vi "Send Get Notifiers.vi"(8 "error in (no error)":errorcluster, 10 "Reply Queue":refnum<queue>, 11 "Message Queue in":refnum<queue>) -> (0 "error out":errorcluster, 3 "Message Queue out":refnum<queue>)   [LabVIEW 2024, in "PID Loop.lvlib" / "Get Notifiers.lvclass"]
uses:
  Get Notifiers.lvclass
  Get Notifiers.lvclass/Get Notifiers.ctl
  C:/Users/uspoaotto/OneDrive - Oregon Tool/Desktop/working copies/helperLoop/src/OOQMH/Message/Message.lvclass
  C:/Users/uspoaotto/OneDrive - Oregon Tool/Desktop/working copies/helperLoop/src/PID Loop/Get Notifiers/Get Notifiers.lvclass
  OOQMH/Message/Message.lvclass
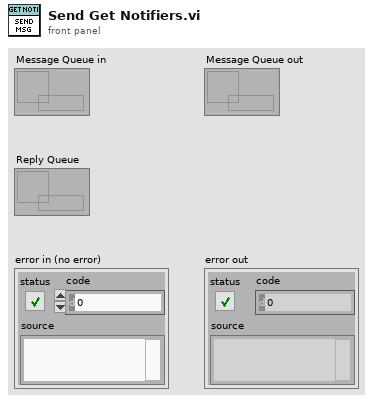
[diagram p1: front panel]
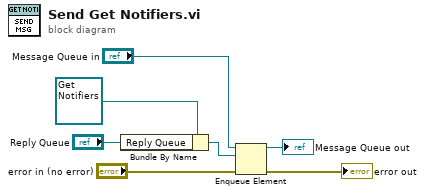
[diagram p0: block diagram]
diagram:
  n1 = Bundle By Name(cluster=refnum<class "Get Notifiers.lvclass"> refnum ("PID Loop.lvlib:Get Notifiers.lvclass"), "Reply Queue"="Reply Queue") -> (w5:refnum<class "Get Notifiers.lvclass">)
  n2 = Enqueue Element(queue="Message Queue in", element=w5, error in (no error)="error in (no error)") -> (queue out=→"Message Queue out":refnum<queue>, error out=→"error out":errorcluster)  [unwired: 1 in, 1 out]
